vi "sendOpenEvent.vi"(8 "error in (no error)":errorcluster, 10 "Path":path, 11 "ScriptEvent in":refnum<class "ScriptEvent.lvclass">) -> (0 "error out":errorcluster, 3 "ScriptEvent out":refnum<class "ScriptEvent.lvclass">)   [LabVIEW 2009, in "Events.lvlib" / "ScriptEvent.lvclass"]
uses:
  ScriptEvent.lvclass
  ScriptEvent.lvclass/ScriptEvent.ctl
  Event.lvclass
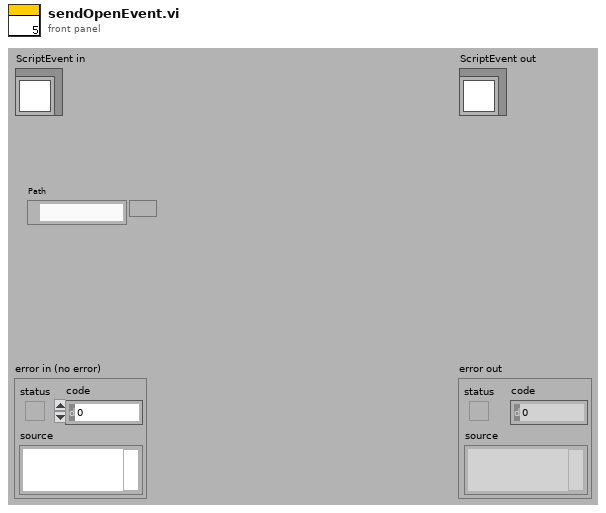
[diagram p1: front panel]
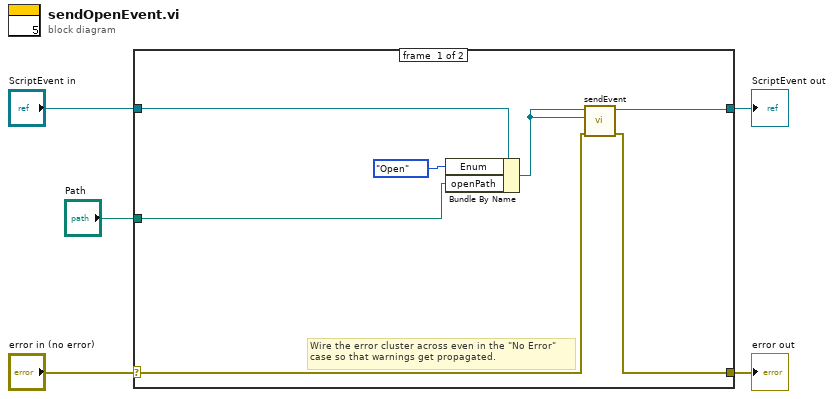
[diagram p0: block diagram]
diagram:
  n1 = case shown="No Error" "error in (no error)" {
    selector: "error in (no error)" -> [w7 w14]
    tunnel: [w6 w14] -> w4
    tunnel: [w9 w13] -> w2
    tunnel: "ScriptEvent in" -> [w10 w13]
    tunnel: "Path" -> [w11 _]
    frame #0 {
      # "Wire the error cluster across even in the \"No Error\"\ncase so that warnings get propagated."
      n2 = Bundle By Name(cluster=w10, "Enum"=enum16{"Open", "Save", "Close"}."Open", "openPath"=w11) -> (w8:refnum<class "ScriptEvent.lvclass">)
      n3 = call "sendEvent.vi"("error in (no error)"=w7, "data"=w8, "Event in"=w8) -> ("error out"=w6:errorcluster, "Event out"=w9:refnum<class "ScriptEvent.lvclass">)  [unwired: 7 in]
    }
    frame #1 {
    }
  }
  "error out" <- w4
  "ScriptEvent out" <- w2
